vi "Disconnect HSD Resources from site.vi"(0 "TSM context":T1, 11 "error in":errorcluster) -> (4 "TSM context out":T1, 15 "error out":errorcluster)   [LabVIEW 2019]
uses:
  <vilib>/NI_TestStand_SemiconductorModule/NI_TestStand_Semiconductor_Module.lvlibp/PinMap/General/SemiconductorModuleContext.ctl
  <instrlib>/niDigital/niDigital.llb/niDigital Selected Function.ctl
  <instrlib>/niDigital/niDigital.llb/niDigital Write Static Pin State.ctl
  <vilib>/NI_TestStand_SemiconductorModule/NI_TestStand_Semiconductor_Module.lvlibp/PinMap/General/NIInstrumentTypeIDs.ctl
  SSC Digital/Configuration/SSC Digital Select Function.vi
  <vilib>/NI_TestStand_SemiconductorModule/NI_TestStand_Semiconductor_Module.lvlibp
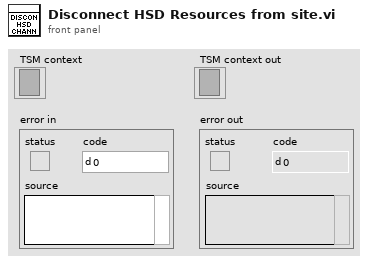
[diagram p1: front panel]
types:
  T1 = typedef "NI_TestStand_Semiconductor_Module.lvlibp/SemiconductorModuleContext.ctl" = refnum<k7>
  T2 = typedef "NI_TestStand_Semiconductor_Module.lvlibp/NIInstrumentTypeIDs.ctl" = string
  T3 = typedef "niDigital Write Static Pin State.ctl" = u8
  T4 = typedef "niDigital Selected Function.ctl" = i32
  T5 = typedef "TSM SSC Digital.ctl" = cluster{"Pin Query Context":refnum<class "DigitalPatternPinQueryContext.lvclass">, "SSC":T6[], "Site Numbers":i32[], "Pins":tag[]}
  T6 = typedef "SSC Digital.ctl" = cluster{"Session":refnum<k15>, "Channel List":string, "Site List":string}
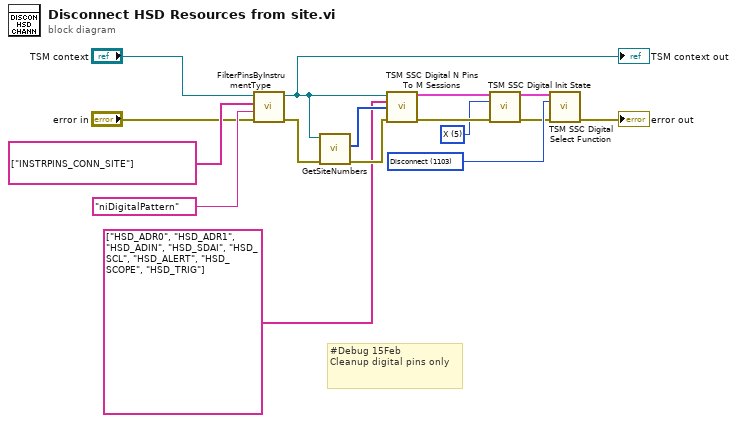
[diagram p0: block diagram]
diagram:
  w12 = T3 5 items=["0"=0, "1"=1, "X"=5] ("state")
  w14 = T4 1103 items=["Digital"=1100, "PPMU"=1101, "Off"=1102, "Disconnect"=1103] ("Select Function")
  # "#Debug 15Feb\nCleanup digital pins only"
  n1 = call <vilib>:"FilterPinsByInstrumentType.vi"("error in (no error)"="error in", "Instrument Type Id"=T2 "niDigitalPattern", "Pins"=string[] ["INSTRPINS_CONN_SITE"], "Semiconductor Module Context"="TSM context") -> ("error out"=w5:errorcluster, "Semiconductor Module Context Out"=w3:T1)  [unwired: 5 in, 1 out]
  "TSM context out" <- w3
  n2 = call <vilib>:"GetSiteNumbers.vi"("error in (no error)"=w5, "Semiconductor Module Context"=w3) -> ("error out"=w4:errorcluster, "Site Numbers"=w2:i32[])  [unwired: 6 in, 2 out]
  n3 = call "TSM SSC Digital N Pins To M Sessions.vi"("TSM context"=w3, "Pins"=tag[] ["HSD_ADR0", "HSD_ADR1", "HSD_ADIN", "HSD_SDAI", "HSD_SCL", "HSD_ALERT", "HSD_SCOPE", "HSD_TRIG"], "Site Numbers"=w2, "error in"=w4) -> ("Digital TSM Out"=w11:T5, "error out"=w16:errorcluster)  [unwired: 10 in]
  n4 = call "TSM SSC Digital Init State.vi"("Digital TSM In"=w11, "state"=w12, "error in"=w16) -> ("Digital TSM Out"=w10:T5, "error out"=w13:errorcluster)  [unwired: 11 in]
  n5 = call "TSM SSC Digital Select Function.vi"("Digital TSM In"=w10, "Function"=w14, "error in"=w13) -> ("error out"=→"error out":errorcluster)  [unwired: 11 in, 1 out]
